vi "New MemberTable.vi"(8 "error in (no error)":errorcluster, 9 "SheetName(\"\")":string, 10 "Path":path, 11 "MemberTable in":refnum<class "TimeTable.lvclass">) -> (0 "error out":errorcluster, 3 "MemberTable out":refnum<class "TimeTable.lvclass">)   [LabVIEW 2015, in "Member_Actor.lvlib" / "TimeTable.lvclass"]
uses:
  TimeTable.lvclass
  TimeTable.lvclass/TimeTable.ctl
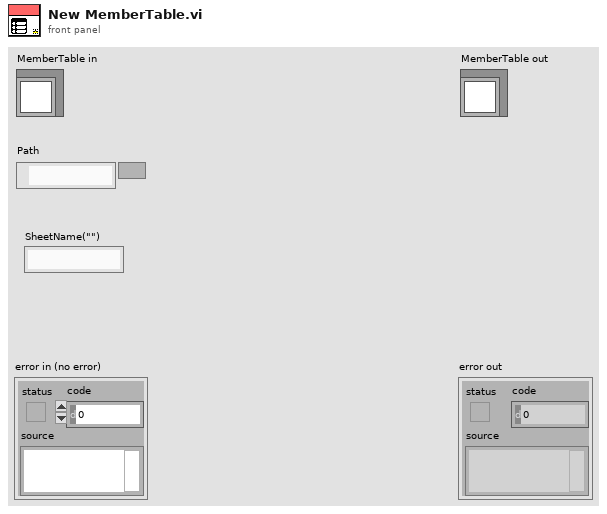
[diagram p1: front panel]
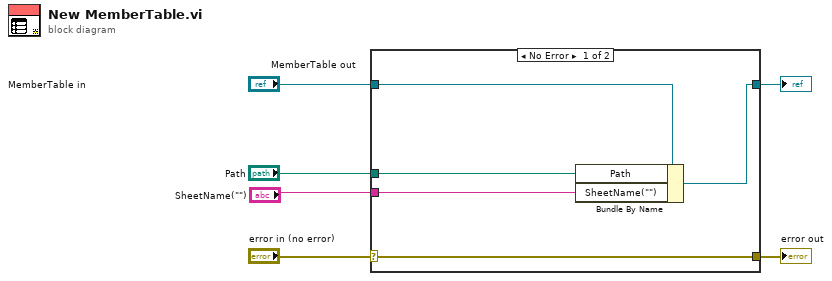
[diagram p0: block diagram]
diagram:
  n1 = case shown="No Error" "error in (no error)" {
    selector: "error in (no error)" -> [w11 w12]
    tunnel: [w11 w12] -> w5
    tunnel: [w9 w13] -> w3
    tunnel: "MemberTable in" -> [w10 w13]
    tunnel: "Path" -> [w8 _]
    tunnel: "SheetName(\"\")" -> [w7 _]
    frame No Error {
      n2 = Bundle By Name(cluster=w10, "Path"=w8, "SheetName(\"\")"=w7) -> (w9:refnum<class "TimeTable.lvclass">)
    }
    frame Error {
    }
  }
  "error out" <- w5
  "MemberTable out" <- w3
